vi "Get Projects.vi"(8 "error in (no error)":errorcluster, 10 "Team GID":string, 11 "Asana in":refnum<class "Asana.lvclass">) -> (0 "error out":errorcluster, 2 "Projects out":T1(array[cluster]), 3 "Asana out":refnum<class "Asana.lvclass">)   [LabVIEW 2016, in "Asana.lvclass"]
uses:
  Asana.lvclass
  Asana.lvclass/Asana.ctl
  <vilib>/addons/_JKI.lib/REST Client/classes/REST Client/REST Client.lvclass
  <vilib>/addons/_JKI.lib/Serialization/JSON/JKI JSON Serialization.lvlib
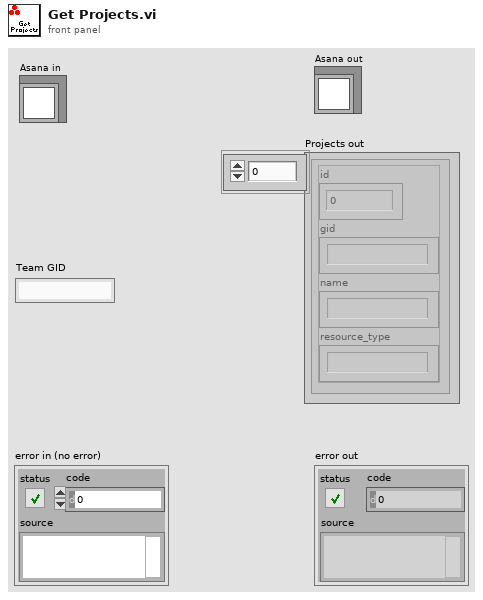
[diagram p1: front panel]
types:
  T1 = cluster{"id":i32, "gid":string, "name":string, "resource_type":string}[]
  T2 = cluster{"data":cluster{"id":i32, "gid":string, "name":string, "resource_type":string}[]}
  T3 = typedef "REST Client.lvlib/REST Client.lvclass/HTTP Header.ctl" = cluster{"header":string, "value":string}
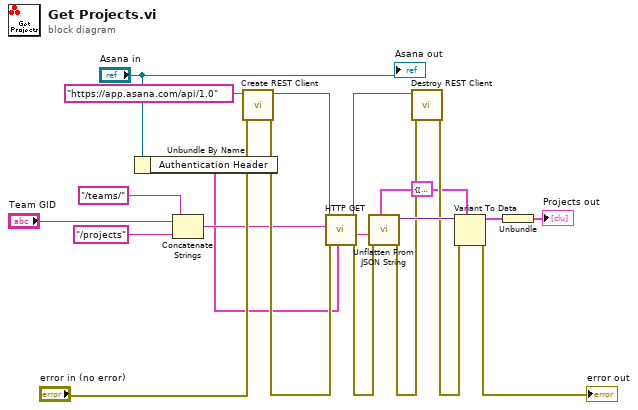
[diagram p0: block diagram]
diagram:
  w6 = T2 {"data"=[{"id"=11111111, "gid"="", "name"="", "resource_type"=""}, {"id"=-3, "gid"="", "name"="", "resource_type"=""}]}
  n1 = Unbundle By Name("Asana in") -> ("Authentication Header"=w1:T3[])
  n2 = Concatenate Strings("/teams/", "Team GID", "/projects" ("Path")) -> (w9:string)
  n3 = call <vilib>:"Create REST Client.vi"("error in (no error)"="error in (no error)", "Base URL"="https://app.asana.com/api/1.0") -> ("error out"=w16:errorcluster, "REST Client out"=w19:refnum<class "REST Client.lvclass">)  [unwired: 8 in]
  n4 = call-dynamic "HTTP GET.vi"("request specific headers"=w1, "error in (no error)"=w16, "Path"=w9, "REST Client in"=w19) -> ("error out"=w13:errorcluster, "Response body"=w14:string, "REST Client out"=w18:refnum<class "REST Client.lvclass">)  [unwired: 2 in, 3 out]
  n5 = call <vilib>:"Unflatten From JSON String.vi"("Type and Defaults"=w6, "error in (no error)"=w13, "JSON String"=w14) -> ("error out"=w12:errorcluster, "Variant"=w15:variant)  [unwired: 7 in]
  n6 = call-dynamic "Destroy REST Client.vi"("error in (no error)"=w12, "REST Client in"=w18) -> ("error out"=w11:errorcluster)  [unwired: 9 in]
  n7 = Variant To Data(error in=w11, type=w6, Variant=w15) -> (data=w5:T2, error out=→"error out":errorcluster)
  n8 = Unbundle(w5) -> ("data"=→"Projects out":T1)
  "Asana out" <- "Asana in"
